vi "Update Signal Selector.vi"(8 "error in (no error)":errorcluster, 11 "Signal Selecton":refnum<vi>) -> (0 "error out":errorcluster)   [LabVIEW 2021, in "Data Analysis.lvlib"]
uses:
  Data Analysis.lvlib
  Support Libraries/Current Value Table/FGVs/Group Memory.vi
  User Interface/User Interface.lvlib
  Support Libraries/Current Value Table/Current Value Table.lvlib
panel:
  in  "Signal Selecton":string[](tree)
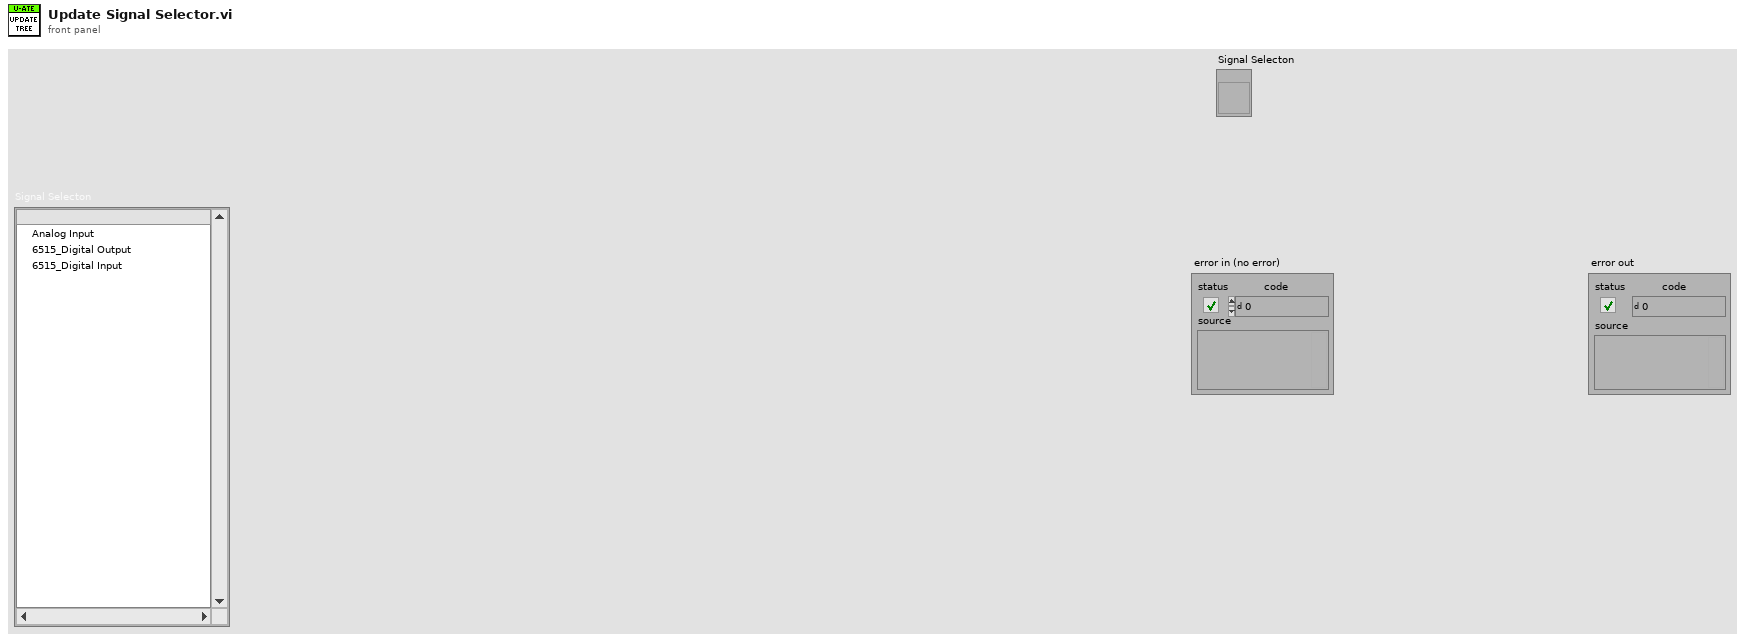
[diagram p1: front panel]
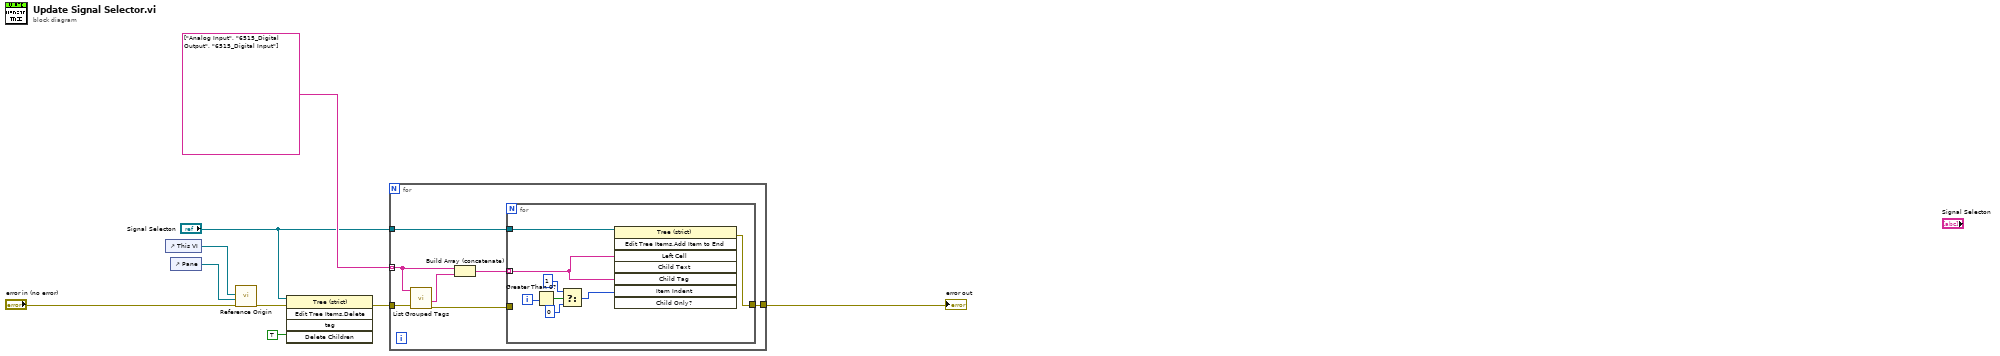
[diagram p0: block diagram]
diagram:
  n1 = control-ref of="This VI"() -> (w9:refnum<vi>)
  n2 = control-ref of="Pane"() -> (w2:refnum<vi>)
  n3 = call "Reference Origin.vi"("error in (no error)"="error in (no error)", "Pane"=w2, "This VI"=w9) -> ("error out"=w8:errorcluster)  [unwired: 8 in]
  n4 = invoke class="Tree (strict)" method="Edit Tree Items.Delete"(reference="Signal Selecton", error in=w8, "Delete Children"=TRUE ("Delete Children?")) -> (error out=w6:errorcluster)  [unwired: 2 in, 4 out]
  n5 = for {
    tunnel: w6 -> [w16]
    tunnel: string[] ["Analog Input", "6515_Digital Output", "6515_Digital Input"] -> [w14] mode=indexing
    tunnel: [w11] -> w3
    tunnel: "Signal Selecton" -> [w10]
    n6 = call "List Grouped Tags.vi"("error in (no error)"=w16, "Group"=w14) -> ("error out"=w15:errorcluster, "Tags Out"=w13:string[])  [unwired: 8 in]
    n7 = Build Array (concatenate)(w14, w13) -> (w12:string[])
    n8 = for {
      tunnel: w15 -> [_]
      tunnel: w12 -> [w19] mode=indexing
      tunnel: [w18] -> w11
      tunnel: w10 -> [w17]
      i -> [w24]
      n9 = Greater Than 0?(x=w24) -> (x > 0?=w23:bool)
      n10 = Select(t=1, s=w23, f=0) -> (s? t:f=w20:i32)
      n11 = invoke class="Tree (strict)" method="Edit Tree Items.Add Item to End"(reference=w17, "Left Cell"=w19, "Child Tag"=w19, "Item Indent"=w20) -> (error out=w18:errorcluster)  [unwired: 4 in, 7 out]
    }
  }
  "error out" <- w3
